vi "Module Cleanup.vi"(8 "error in (no error)":errorcluster, 11 "Volatus Core in":refnum<class "Volatus Core.lvclass">) -> (0 "error out":errorcluster, 3 "Volatus Core out":refnum<class "Volatus Core.lvclass">)   [LabVIEW 2020, in "Volatus.lvlib" / "Volatus Core.lvclass"]
uses:
  Volatus Core.lvclass
  Module/Module.lvclass/Module.ctl
  Volatus Core.lvclass/Volatus Core.ctl
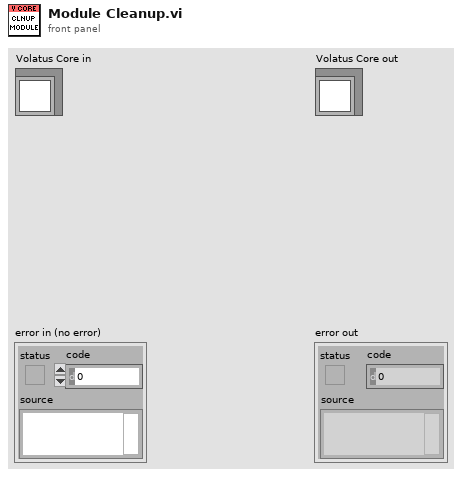
[diagram p1: front panel]
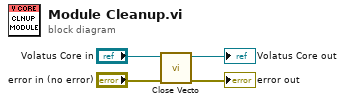
[diagram p0: block diagram]
diagram:
  n1 = call "Close Vecto.vi"("error in (no error)"="error in (no error)", "Volatus Core in"="Volatus Core in") -> ("error out"=→"error out":errorcluster, "Volatus Core out"=→"Volatus Core out":refnum<class "Volatus Core.lvclass">)  [unwired: 8 in]
